vi "FireVI_1.vi"() -> ()   [LabVIEW 2011]
uses:
  UserEvent.ctl
panel:
  in  "UserEvent":T1
  in  "stop":bool
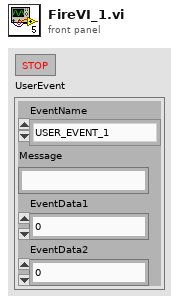
[diagram p1: front panel]
types:
  T1 = typedef "UserEvent.ctl" = cluster{"EventName":enum16{"USER_EVENT_1", "USER_EVENT_2", "USER_EVENT_3", "USER_EVENT_4", "USER_EVENT_5", "USER_EVENT_6", "USER_EVENT_7", "USER_EVENT_8", "USER_EVENT_9", "USER_EVENT_10"}, "Message":string, "EventData1":dbl, "EventData2":dbl}
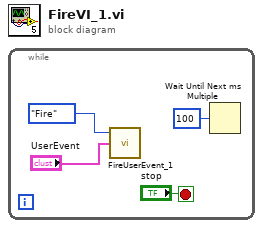
[diagram p0: block diagram]
diagram:
  n1 = while {
    stop <- "stop" stop-if-true
    n2 = call "FireUserEvent_1.vi"("UserEvent"="UserEvent", "Enum"=enum16{"GetRef", "Fire", "Release"}."Fire") -> ()  [unwired: 1 in, 2 out]
    n3 = Wait Until Next ms Multiple(millisecond multiple=u32 100) -> ()  [unwired: 1 out]
  }
